vi "Verbindung herstellen.vi"(8 "error in (no error)":errorcluster caption="Fehler (Eingang, kein Fehler)", 10 "IP Adresse":string="192.168.15.101", 11 "Steuerung PNS (Eingang)":refnum<class "Steuerung PNS.lvclass">) -> (0 "error out":errorcluster caption="Fehler (Ausgang)", 3 "Steuerung PNS (Ausgang)":refnum<class "Steuerung PNS.lvclass">)   [LabVIEW 2020, in "Steuerung PNS.lvclass"]
doc: "Stellt eine Modbus Verbindung mit der angegebenen IP Adresse her,\nund fragt die Kennung der Steuerungs Type ab. \nDaraus wird dann die jeweilige SubKlasse erzeugt und als transparente SteuerungsKlasse wieder zurück gegeben.\nDie Modbus Referenz wird im Objekt gespeichert.\nRIW"
uses:
  Steuerung PNS.lvclass
  Steuerung PNS.lvclass/Steuerung PNS.ctl
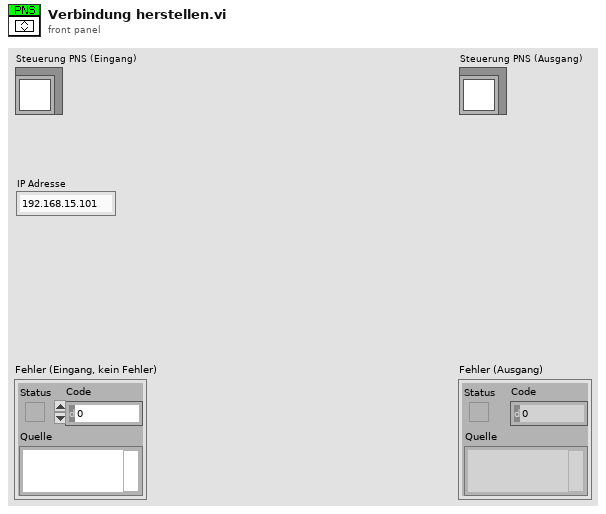
[diagram p1: front panel]
types:
  T1 = typedef "Steuerung PNS.lvclass/Adresse.ctl" = cluster{i32[][], i32}
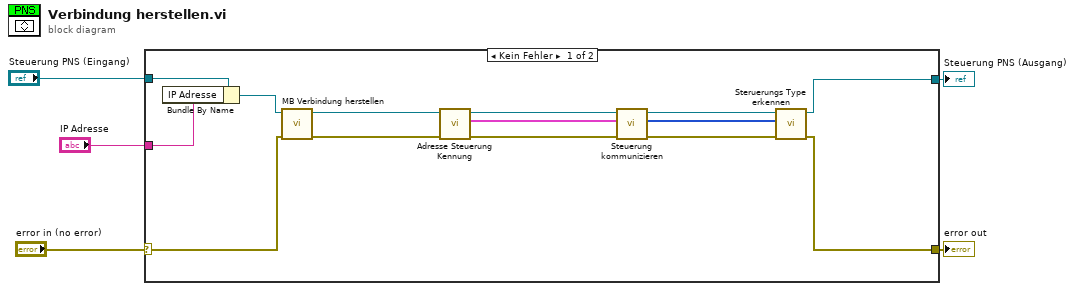
[diagram p0: block diagram]
diagram:
  n1 = case shown="Kein Fehler" "error in (no error)" {
    selector: "error in (no error)" -> [w15 w20]
    tunnel: [w13 w20] -> w4
    tunnel: [w16 w21] -> w2
    tunnel: "Steuerung PNS (Eingang)" -> [w19 w21]
    tunnel: "IP Adresse" -> [w11 _]
    frame No Error {
      n2 = Bundle By Name(cluster=w19, "IP Adresse"=w11) -> (w12:refnum<class "Steuerung PNS.lvclass">)
      n3 = call "MB Verbindung herstellen.vi"("error in (no error)"=w15, "Steuerung PNS Eingang"=w12) -> ("error out"=w8:errorcluster, "Steuerung PNS Ausgang"=w9:refnum<class "Steuerung PNS.lvclass">)  [unwired: 8 in]
      n4 = call "Adresse Steuerung Kennung.vi"("error in (no error)"=w8, "Steuerung PNS Eingang"=w9) -> ("error out"=w7:errorcluster, "Adressen"=w6:T1, "Steuerung PNS Ausgang"=w10:refnum<class "Steuerung PNS.lvclass">)  [unwired: 7 in]
      n5 = call "Steuerung kommunizieren.vi"("Steuerung PNS Eingang"=w10, "Adressen"=w6, "error in (no error)"=w7) -> ("Steuerung PNS Ausgang"=w18:refnum<class "Steuerung PNS.lvclass">, "Istwerte"=w17:u16[], "error out"=w14:errorcluster)  [unwired: 5 in]
      n6 = call "Steruerungs Type erkennen.vi"("error in (no error)"=w14, "Steuerungs Type"=w17, "Steuerung PNS Eingang"=w18) -> ("error out"=w13:errorcluster, "Steuerung PNS Ausgang"=w16:refnum<class "Steuerung PNS.lvclass">)  [unwired: 7 in]
    }
    frame Error {
    }
  }
  "error out" <- w4
  "Steuerung PNS (Ausgang)" <- w2
